vi "Write Sideways Synced Motors.vi"(8 "error in (no error)":errorcluster, 10 "Actor Framework:Message Enqueuer":refnum<class "Message Enqueuer.lvclass">, 11 "Sideways Drive in":refnum<class "Sideways Drive.lvclass">) -> (0 "error out":errorcluster, 3 "Sideways Drive out":refnum<class "Sideways Drive.lvclass">)   [LabVIEW 2014, in "Sideways Drive.lvlib" / "Sideways Drive.lvclass"]
uses:
  Sideways Drive.lvclass
  <vilib>/ActorFramework/Message Enqueuer/Message Enqueuer.lvclass
  Sideways Drive.lvclass/Sideways Drive.ctl
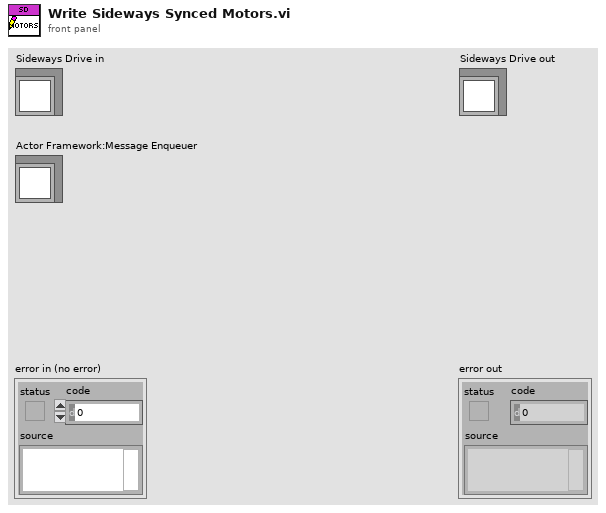
[diagram p1: front panel]
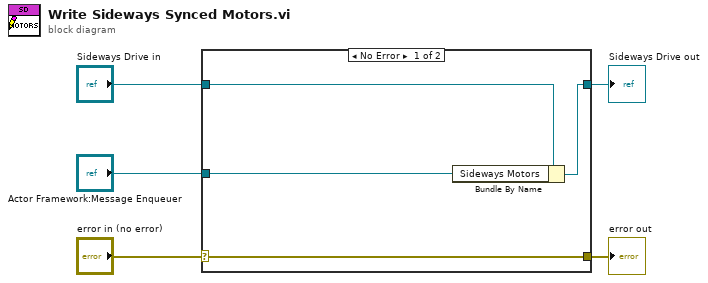
[diagram p0: block diagram]
diagram:
  n1 = case shown="No Error" "error in (no error)" {
    selector: "error in (no error)" -> [w9 w10]
    tunnel: [w9 w10] -> w4
    tunnel: [w7 w11] -> w2
    tunnel: "Sideways Drive in" -> [w8 w11]
    tunnel: "Actor Framework:Message Enqueuer" -> [w6 _]
    frame No Error {
      n2 = Bundle By Name(cluster=w8, "Sideways Motors"=w6) -> (w7:refnum<class "Sideways Drive.lvclass">)
    }
    frame Error {
    }
  }
  "error out" <- w4
  "Sideways Drive out" <- w2
